vi "Decimate.vi"   [LabVIEW 2019, in "xy_utilities.lvlib"]
doc: "Decimates the X and Y arrays of the input XY-data by the chosen decimating factor and the averaging controls. \n\nWire data to the data inputs to determine the polymorphic instance to use or manually select the instance."
uses:
  xy_utilities.lvlib
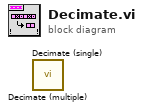
[diagram p0: block diagram]
diagram:
  n1 = call "Decimate (multiple).vi"() -> ()  [unwired: 10 in, 2 out]
  n2 = call "Decimate (single).vi"() -> ()  [unwired: 10 in, 2 out]
